vi "Teleop.vi"(10 "Match Info":T2={"Autonomous Elapsed Seconds"=0.0, "TeleOp Elapsed Seconds"=0.0, "Disabled Elapsed Seconds"=0.0, "Visited Autonomous"=FALSE, "Visited TeleOp"=FALSE, "Visited Disabled"=FALSE, "Autonomous Settings"={"Autonomous Style"=enum."Independent", "VI Refnum"=refnum}}, 11 "Call Context":T3) -> ()   [LabVIEW 2019]
doc: "This VI is called for each TeleOp packet received from the DS where the robot is not disabled. It is often used to read from the joysticks and update I/O or to update setpoints for timed control loops. It should complete and return within 20 milliseconds or it may miss DS packets."
uses:
  <vilib>/Rock Robotics/WPI/DriverStation/WPI_DriverStationDerivedRobotMode.ctl
  <vilib>/Rock Robotics/WPI/DriverStation/WPI_DriverStationMatch Info.ctl
  <vilib>/Rock Robotics/WPI/ThirdParty/REV Robotics/SPARK MAX/Typedef/Spark MAX Control Type.ctl
  <vilib>/Rock Robotics/WPI/Utilities/WPI_GetSetVariantRefNum.vi
  <vilib>/Rock Robotics/Network Tables/NT Write Boolean Array.vi
  <vilib>/Rock Robotics/Network Tables/NT Write Numeric Array.vi
  <vilib>/Rock Robotics/Network Tables/NT Read Boolean.vi
  <vilib>/Rock Robotics/Network Tables/NT Read Number.vi
  <vilib>/Rock Robotics/Network Tables/NT Write Number.vi
  Robot Global Data.vi
panel:
  in  "lower percent":dbl=0.62
  out "lower Velocity":dbl
  out "Waveform Chart":T1(graph)
  in  "top percent":dbl=0.33
  out "top Velocity":dbl
  out "Sample Slider 0":dbl(slide) scale=0.0..5.0
  out "Sample Boolean 1":bool
  out "Sample Boolean 0":bool
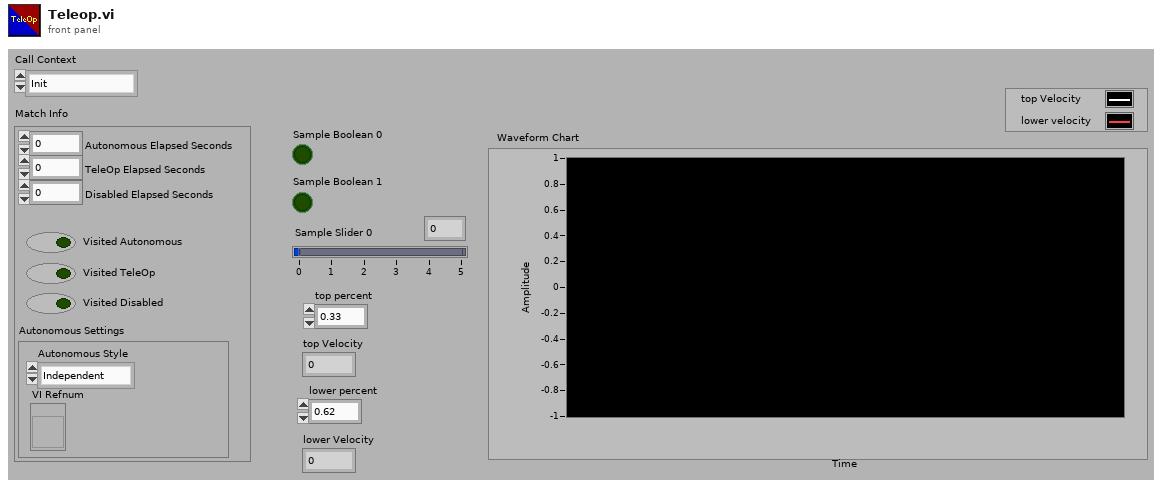
[diagram p1: front panel]
types:
  T1 = cluster{"Sensor Velocity":dbl, "Sensor Velocity":dbl}
  T2 = typedef "WPI_DriverStationMatch Info.ctl" = cluster{"Autonomous Elapsed Seconds":dbl, "TeleOp Elapsed Seconds":dbl, "Disabled Elapsed Seconds":dbl, "Visited Autonomous":bool, "Visited TeleOp":bool, "Visited Disabled":bool, "Autonomous Settings":cluster{"Autonomous Style":enum16{"Iterative", "Independent"}, "VI Refnum":refnum<vi>}}
  T3 = typedef "WPI_DriverStationDerivedRobotMode.ctl" = enum16{"Init", "Execute", "Stop"}
  T4 = typedef "Spark MAX Control Type.ctl" = enum16{"Percent VBus", "Voltage", "Velocity", "Position", "Smart Motion", "Current", "Smart Velocity"}
  T5 = typedef "WPI_JoystickDevRef.ctl" = cluster{"Device":T6}
  T6 = typedef "WPI_JoystickDeviceEnum.ctl" = enum16{"USB 0", "USB 1", "USB 2", "USB 3", "USB 4", "USB 5"}
  T7 = typedef "WPI_RobotDriveDevRef.ctl" = cluster{"DevStatus":errorcluster, "Motors[]":T8[], "Square Inputs":bool, "Max Output":dbl}
  T8 = typedef "WPI_MotorControlDeviceRef.ctl" = cluster{"DeviceStatus":errorcluster, "Type":T9, "PWM":cluster{"PWM Channel":T10, "DeadBand":T11}, "CAN":cluster{"Device Number":u8, "SetOutput VI Ref":variant, "GetOutput VI Ref":variant, "Enable VI Ref":variant, "Disable VI Ref":variant, "Data":variant}, "Invert":bool, "DIO PWM":cluster{"PWM \"Enable\" Channel":T10, "DIOChannel":T12, "PWM Rate":dbl}}
  T9 = typedef "WPI_MotorControlType.ctl" = enum16{"PWM", "CAN", "DIO PWM"}
  T10 = typedef "FPGA_DIOPWMChannel.ctl" = enum8{"PWM 0", "PWM 1", "PWM 2", "PWM 3", "PWM 4", "PWM 5", "PWM 6", "PWM 7", "PWM 8", "PWM 9", "PWM MXP 0", "PWM MXP 1", "PWM MXP 2", "PWM MXP 3", "PWM MXP 4", "PWM MXP 5", "PWM MXP 6", "PWM MXP 7", "PWM MXP 8", "PWM MXP 9", "Invalid"}
  T11 = typedef "WPI_PWMDeadband.ctl" = cluster{"Name":string, "maxPositivePwm":i32, "minPositivePwm":i32, "centerPwm":i32, "maxNegativePwm":i32, "minNegativePwm":i32, "angularRange":u16}
  T12 = typedef "FPGA_DIOChannel.ctl" = enum8{"DIO 0", "DIO 1", "DIO 2", "DIO 3", "DIO 4", "DIO 5", "DIO 6", "DIO 7", "DIO 8", "DIO 9", "DIO MXP 0", "DIO MXP 1", "DIO MXP 2", "DIO MXP 3", "DIO MXP 4", "DIO MXP 5", "DIO MXP 6", "DIO MXP 7", "DIO MXP 8", "DIO MXP 9", "DIO MXP 10", "DIO MXP 11", "DIO MXP 12", "DIO MXP 13", "DIO MXP 14", "DIO MXP 15", "SPI Port CS1", "SPI Port CS2", "SPI Port CS3", "SPI Port MISO", "SPI Port MOSI", "Invalid"}
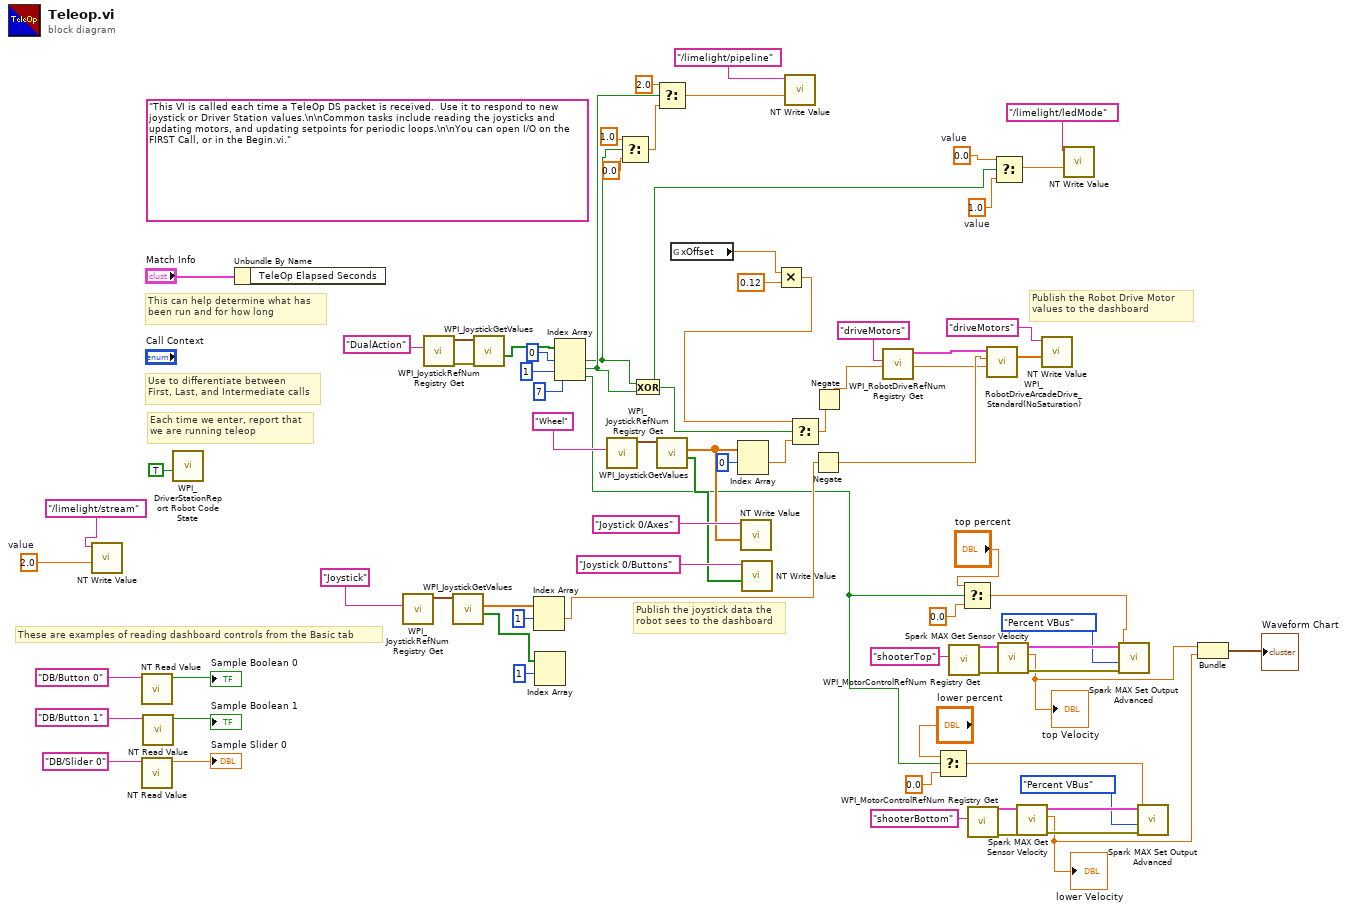
[diagram p0: block diagram]
diagram:
  w13 = 2.0  # value
  w19 = 0.0  # value
  w21 = 1.0  # value
  (unwired) "This VI is called each time a TeleOp DS packet is received.  Use it to respond to new joystick or Driver Station values.\n\nCommon tasks include reading the joysticks and updating motors, and updating setpoints for periodic loops.\n\nYou can open I/O on the FIRST Call, or in the Begin.vi."
  # "Publish the Robot Drive Motor\nvalues to the dashboard"
  # "These are examples of reading dashboard controls from the Basic tab"
  # "Publish the joystick data the\nrobot sees to the dashboard"
  # "Each time we enter, report that\nwe are running teleop"
  # "Use to differentiate between\nFirst, Last, and Intermediate calls"
  # "This can help determine what has\nbeen run and for how long"
  n1 = call-poly <vilib>:"NT Write Value.vi"("Numeric"=w13, "Name"="/limelight/stream") -> ()  [unwired: 9 in, 1 out]
  n2 = call-poly <vilib>:"NT Read Value.vi"("Name"="DB/Button 0" ("refnum name")) -> ("Boolean"=→"Sample Boolean 0":bool)  [unwired: 9 in, 1 out]
  n3 = call-poly <vilib>:"NT Read Value.vi"("Name"="DB/Slider 0" ("refnum name")) -> ("Numeric"=→"Sample Slider 0":dbl)  [unwired: 9 in, 1 out]
  n4 = call-poly <vilib>:"NT Read Value.vi"("Name"="DB/Button 1" ("refnum name")) -> ("Boolean"=→"Sample Boolean 1":bool)  [unwired: 9 in, 1 out]
  n5 = call <vilib>:"WPI_DriverStationReport Robot Code State.vi"("TeleOp"=TRUE ("Autonomous")) -> ()  [unwired: 10 in, 1 out]
  n6 = Unbundle By Name("Match Info") -> ()  [unwired: 1 out]
  n7 = call <vilib>:"WPI_JoystickRefNum Registry Get.vi"("refnum name"="Joystick") -> ("JoystickDevRef"=w63:T5)  [unwired: 1 in, 9 out]
  n8 = call <vilib>:"WPI_JoystickRefNum Registry Get.vi"("refnum name"="DualAction") -> ("error out"=w35:errorcluster, "JoystickDevRef"=w38:T5)  [unwired: 1 in, 8 out]
  n9 = call <vilib>:"WPI_JoystickGetValues.vi"("JoystickDevRef"=w63) -> ("Buttons"=w1:bool[], "Axes"=w62:dbl[])  [unwired: 6 in, 3 out]
  n10 = call <vilib>:"WPI_JoystickGetValues.vi"("error in (no error)"=w35, "JoystickDevRef"=w38) -> ("Buttons"=w34:bool[])  [unwired: 5 in, 4 out]
  n11 = Index Array(array=w62, index #1=1 ("index")) -> (element #1=w30:dbl)  [unwired: 1 in, 1 out]
  n12 = Index Array(array=w1, index #1=1 ("index")) -> ()  [unwired: 1 in, 2 out]
  n13 = Index Array(array=w34, index #1=0 ("index"), index #2=1 ("index"), index #3=7 ("index")) -> (element #1=w9:bool, element #2=w18:bool, element #3=w26:bool)
  n14 = call <vilib>:"WPI_JoystickRefNum Registry Get.vi"("refnum name"="Wheel") -> ("JoystickDevRef"=w75:T5)  [unwired: 1 in, 9 out]
  n15 = Select(t=1.0 ("f"), s=w9, f=0.0) -> (s? t:f=w8:dbl)
  n16 = Exclusive Or(1:w18, 2:w9) -> (0:w14:bool)
  n17 = Select(t=2.0, s=w18, f=w8) -> (s? t:f=w23:dbl)
  n18 = call <vilib>:"WPI_JoystickGetValues.vi"("JoystickDevRef"=w75) -> ("Buttons"=w53:bool[], "Axes"=w71:dbl[])  [unwired: 6 in, 3 out]
  n19 = global read "Robot Global Data.vi" "xOffset"() -> (w17:dbl)
  n20 = Index Array(array=w71, index #1=0 ("index")) -> (element #1=w39:dbl)  [unwired: 1 in, 1 out]
  n21 = call-poly <vilib>:"NT Write Value.vi"("Numeric Array"=w71, "Name"="Joystick 0/Axes") -> ()  [unwired: 9 in, 1 out]
  n22 = call-poly <vilib>:"NT Write Value.vi"("Boolean Array"=w53, "Name"="Joystick 0/Buttons") -> ()  [unwired: 9 in, 1 out]
  n23 = Multiply(x=w17, y=0.12) -> (x*y=w15:dbl)
  n24 = call-poly <vilib>:"NT Write Value.vi"("Numeric"=w23, "Name"="/limelight/pipeline") -> ()  [unwired: 9 in, 1 out]
  n25 = Select(t=w15, s=w14, f=w39) -> (s? t:f=w31:dbl)
  n26 = Negate(x=w30) -> (-x=w29:dbl)
  n27 = Negate(x=w31) -> (-x=w7:dbl)
  n28 = call <vilib>:"WPI_RobotDriveRefNum Registry Get.vi"("refnum name"="driveMotors") -> ("RobotDriveDevRef"=w5:T7)  [unwired: 1 in, 9 out]
  n29 = Select(t="lower percent", s=w26, f=0.0) -> (s? t:f=w42:dbl)
  n30 = call <vilib>:"WPI_MotorControlRefNum Registry Get.vi"("refnum name"="shooterTop") -> ("error out"=w54:errorcluster, "MotorControlDevRef"=w55:T8)  [unwired: 9 in]
  n31 = Select(t="top percent", s=w26, f=0.0) -> (s? t:f=w40:dbl)
  n32 = call <vilib>:"WPI_MotorControlRefNum Registry Get.vi"("refnum name"="shooterBottom") -> ("error out"=w46:errorcluster, "MotorControlDevRef"=w47:T8)  [unwired: 9 in]
  n33 = call <vilib>:"WPI_RobotDriveArcadeDrive_Standard(NoSaturation).vi"("Y axis value"=w7, "X axis value"=w29, "RobotDriveDevRef"=w5) -> ("Motor Values"=w4:dbl[])  [unwired: 1 in, 7 out]
  n34 = Select(t=w19, s=w14, f=w21) -> (s? t:f=w20:dbl)
  n35 = call <vilib>:"Spark MAX Get Sensor Velocity.vi"("error in (no error)"=w54, "MotorControlDevRef in"=w55) -> ("error out"=w57:errorcluster, "Sensor Velocity"=w52:dbl, "MotorControlDevRef out"=w58:T8)  [unwired: 6 in, 1 out]
  "top Velocity" <- w52
  n36 = call <vilib>:"Spark MAX Get Sensor Velocity.vi"("error in (no error)"=w46, "MotorControlDevRef in"=w47) -> ("error out"=w49:errorcluster, "Sensor Velocity"=w28:dbl, "MotorControlDevRef out"=w50:T8)  [unwired: 6 in, 1 out]
  "lower Velocity" <- w28
  n37 = call-poly <vilib>:"NT Write Value.vi"("Numeric Array"=w4, "Name"="driveMotors") -> ()  [unwired: 9 in, 1 out]
  n38 = call-poly <vilib>:"NT Write Value.vi"("Numeric"=w20, "Name"="/limelight/ledMode") -> ()  [unwired: 9 in, 1 out]
  n39 = call <vilib>:"Spark MAX Set Output Advanced.vi"("error in (no error)"=w57, "Control Mode"=Spark_MAX_Control_Type."Percent VBus", "Setpoint"=w40, "MotorControlDevRef"=w58) -> ()  [unwired: 6 in, 2 out]
  n40 = call <vilib>:"Spark MAX Set Output Advanced.vi"("error in (no error)"=w49, "Control Mode"=Spark_MAX_Control_Type."Percent VBus", "Setpoint"=w42, "MotorControlDevRef"=w50) -> ()  [unwired: 6 in, 2 out]
  n41 = Bundle("Sensor Velocity"=w52, "Sensor Velocity"=w28) -> (→"Waveform Chart":T1)  [unwired: 1 in]
